vi "Read Keyboard Action Type.vi"(8 "error in (no error)":errorcluster, 11 "Keyboard Action in":refnum<class "Keyboard Action.lvclass">) -> (0 "error out":errorcluster, 2 "Keyboard Action Type":T1, 3 "Keyboard Action out":refnum<class "Keyboard Action.lvclass">)   [LabVIEW 2020, in "MacroAssert.lvlib" / "Keyboard Action.lvclass"]
uses:
  Keyboard Action.lvclass
  Keyboard Action Type.ctl
  Keyboard Action.lvclass/Keyboard Action.ctl
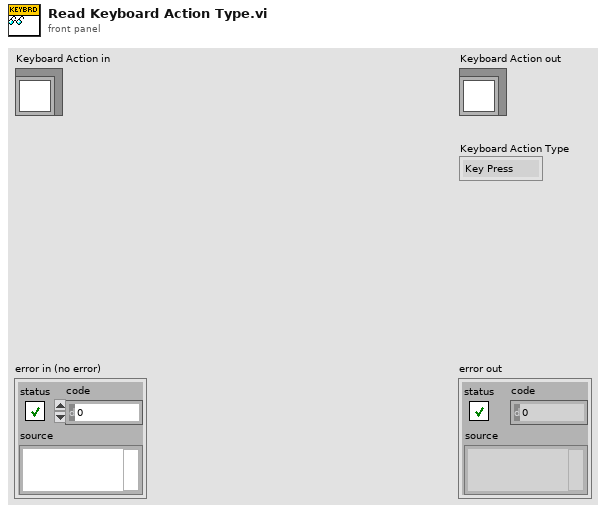
[diagram p1: front panel]
types:
  T1 = typedef "MacroAssert.lvlib/Keyboard Action.lvclass/Keyboard Action Type.ctl" = enum16{"Key Press", "Key Down", "Key Up"}
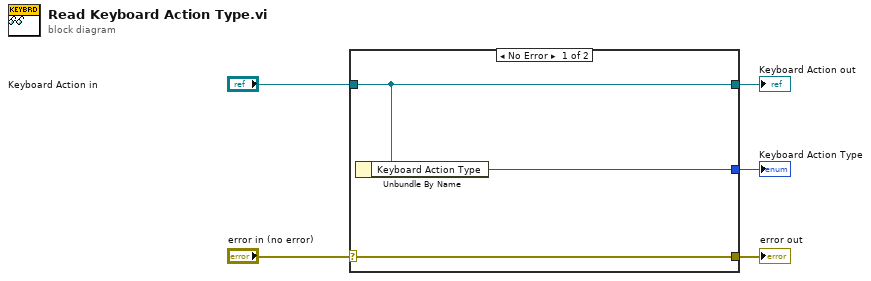
[diagram p0: block diagram]
diagram:
  n1 = case shown="No Error" "error in (no error)" {
    selector: "error in (no error)" -> [w8 w9]
    tunnel: [w8 w9] -> w4
    tunnel: [w7 w10] -> w2
    tunnel: "Keyboard Action in" -> [w7 w10]
    tunnel: [w6 _] -> w1
    frame No Error {
      n2 = Unbundle By Name(w7) -> ("Keyboard Action Type"=w6:T1)
    }
    frame Error {
    }
  }
  "error out" <- w4
  "Keyboard Action out" <- w2
  "Keyboard Action Type" <- w1
